vi "Read Saturator Temperature.vi"(8 "error in":errorcluster, 11 "3010 in":refnum<class "3010.lvclass">) -> (0 "error out":errorcluster, 2 "satT":sgl, 3 "3010 out":refnum<class "3010.lvclass">)   [LabVIEW 2014, in "3010.lvclass"]
doc: "Get the saturator temperature from the 3010 CPC."
uses:
  3010.lvclass
  Controls/CmdStruct.ctl
  Controls/Enum Cmd.ctl
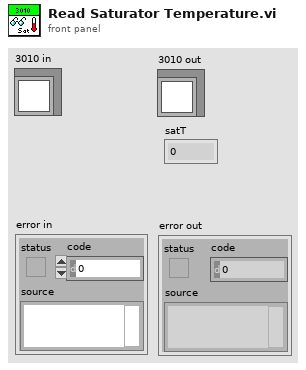
[diagram p1: front panel]
types:
  T1 = typedef "3010.lvclass/Enum Cmd.ctl" = enum16{"Dump", "Dump Cumulative", "Read Liquid Status", "Read Condenser Temperature", "Read Saturator Temperature", "Read Environment", "Read 6 s Buffer", "Read 1 s Buffer", "Read Concentration Display", "Read Delta T", "Read Vacuum Status", "Set Analog Voltage", "Execute Fill", "Clear Display Buffers"}
  T2 = typedef "CmdStruct.ctl" = cluster{"Cmd":u8, "x":i64, "y":i64, "Display":string}
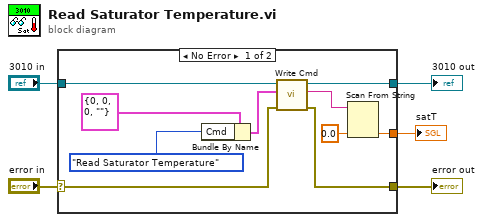
[diagram p0: block diagram]
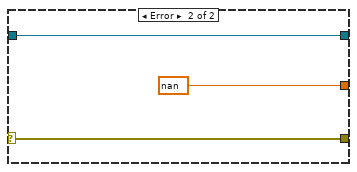
[diagram p2: hidden frame]
diagram:
  n1 = case shown="No Error" "error in" {
    selector: "error in" -> [w13 w18]
    tunnel: [w9 w18] -> w4
    tunnel: [w10 w17] -> w2
    tunnel: "3010 in" -> [w15 w17]
    tunnel: [w6 sgl nan ("default value 1")] -> w1
    frame No Error {
      n2 = Bundle By Name(cluster=T2 {"Cmd"=0, "x"=0, "y"=0, "Display"=""} ("CmdStruct"), "Cmd"=Enum_Cmd."Read Saturator Temperature" ("Enum Cmd")) -> (w11:T2)
      n3 = call-dynamic "Write Cmd.vi"("error in"=w13, "CmdStruct"=w11, "CPC in"=w15) -> ("error out"=w9:errorcluster, "Buffer"=w8:string, "CPC out"=w10:refnum<class "3010.lvclass">)  [unwired: 6 in]
      n4 = Scan From String(input string=w8, default 1=sgl 0.0 ("default value 1")) -> (output 1=w6:sgl)  [unwired: 3 in, 3 out]
    }
    frame Error {
    }
  }
  "error out" <- w4
  "3010 out" <- w2
  "satT" <- w1
